vi "ReadSerial.vi"(8 "error in (no error)":errorcluster, 11 "VISA Refnum in":refnum<visa-resource-name>) -> (0 "error out":errorcluster, 2 "String":string, 3 "VISA Refnum out":refnum<visa-resource-name>)   [LabVIEW 2019]
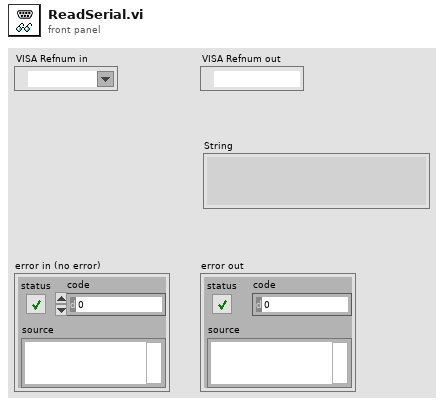
[diagram p1: front panel]
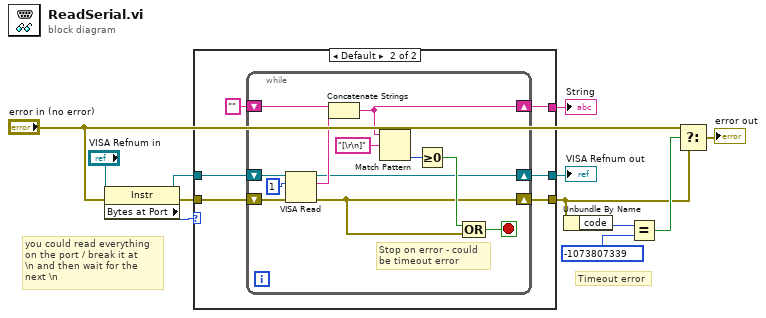
[diagram p0: block diagram]
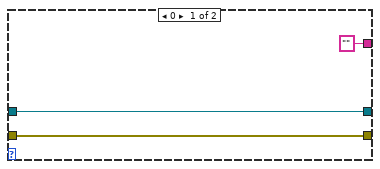
[diagram p2: hidden frame]
diagram:
  # "Timeout error"
  # "you could read everything\non the port / break it at\n\\n and then wait for the\nnext \\n"
  n1 = property class="Instr"(reference="VISA Refnum in", error in="error in (no error)") -> (reference out=w8:refnum<visa-resource-name>, error out=w10:errorcluster, "Bytes at Port"=w12:u32)
  n2 = case shown="Default" w12 {
    tunnel: w8 -> [w15 w21]
    tunnel: w10 -> [w14 w20]
    tunnel: [w14 w19] -> w2
    tunnel: [w15 w18] -> w11
    tunnel: ["" w16] -> w7
    frame 0 {
    }
    frame Default {
      n3 = while {
        shift-right: [w23] -> w18
        shift-left: w21 -> [w33]
        shift-right: [w22] -> w19
        shift-left: w20 -> [w32]
        shift-right: [w28] -> w16
        shift-left: "" -> [w30]
        stop <- w24 stop-if-true
        # "Stop on error - could\nbe timeout error"
        n4 = VISA Read(VISA resource name=w33, byte count=u32 1, error in (no error)=w32) -> (VISA resource name out=w23:refnum<visa-resource-name>, read buffer=w29:string, error out=w22:errorcluster)  [unwired: 1 out]
        n5 = Concatenate Strings(w30, w29) -> (w28:string)
        n6 = Match Pattern(string=w28, regular expression="[\r\n]") -> (offset past match=w26:i32)  [unwired: 1 in, 3 out]
        n7 = Greater Or Equal To 0?(x=w26) -> (x >= 0?=w25:bool)
        n8 = Compound Arithmetic op=OR(w25, w22) -> (w24:bool)
      }
    }
  }
  "VISA Refnum out" <- w11
  "String" <- w7
  n9 = Unbundle By Name(w2) -> ("code"=w6:i32)
  n10 = Equal?(x=w6, y=-1073807339 ("code")) -> (x = y?=w4:bool)
  n11 = Select(t="error in (no error)", s=w4, f=w2) -> (s? t:f=→"error out":errorcluster)
